vi "Tosca-Test for End of Block.vi"(0 "Result":T1, 1 "SCL in":T2[](array[typedef]), 2 "StimCon Element":T2, 9 "sclIndex":i32, 11 "error in (no error)":errorcluster, 12 "Ncomplete":i32, 13 "Abort":bool) -> (3 "SCL out":T2[](array[typedef]), 4 "Result thru":T1, 6 "End block?":bool, 8 "Abort?":bool, 14 "Ncomplete out":i32, 15 "error out":errorcluster)   [LabVIEW 2020]
uses:
  Typedefs/Tosca-SCL Element.ctl
  Typedefs/Tosca-Schedule Mode.ctl
  Typedefs/Tosca-Event Type.ctl
  Typedefs/Tosca-Trial Result Enum.ctl
  Tosca-Globals.vi
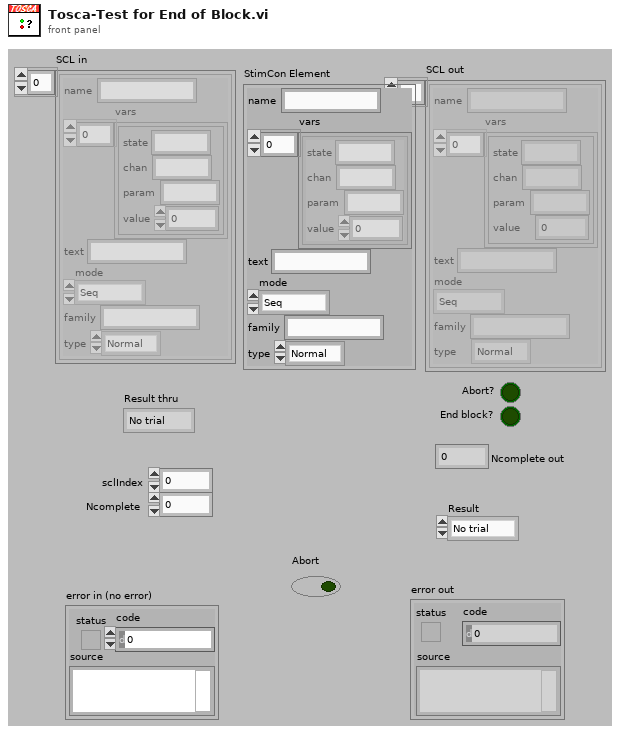
[diagram p1: front panel]
types:
  T1 = typedef "Tosca-Trial Result Enum.ctl" = enum16{"No trial", "Go", "No go", "Error", "Abort"}
  T2 = typedef "Tosca-SCL Element.ctl" = cluster{"name":string, "vars":cluster{"state":string, "chan":string, "param":string, "value":dbl}[], "text":string, "mode":T3, "family":string, "type":T4}
  T3 = typedef "Tosca-Schedule Mode.ctl" = enum16{"Seq", "CS+/CS-", "Adapt"}
  T4 = typedef "Tosca-Event Type.ctl" = enum16{"Normal", "CS+", "CS-"}
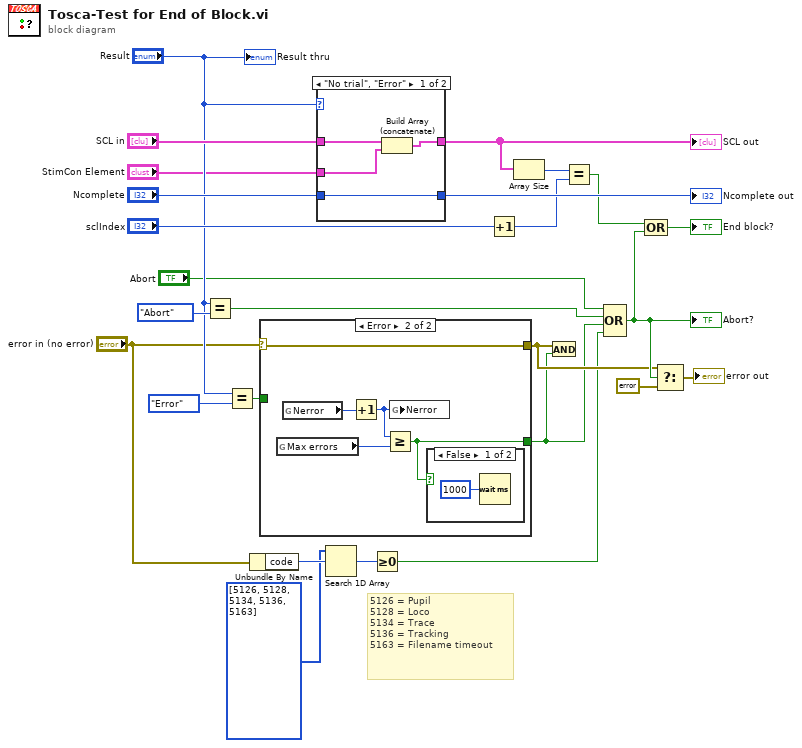
[diagram p0: block diagram]
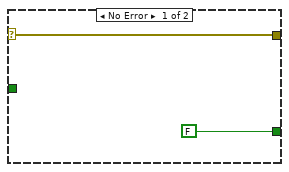
[diagram p2: hidden frame]
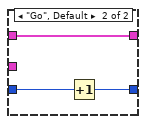
[diagram p4: hidden frame]
diagram:
  # "5126 = Pupil\n5128 = Loco\n5134 = Trace\n5136 = Tracking\n5163 = Filename timeout"
  n1 = Equal?(x="Result", y=Tosca-Trial_Result_Enum."Abort") -> (x = y?=w13:bool)
  n2 = Equal?(x="Result", y=Tosca-Trial_Result_Enum."Error") -> (x = y?=w10:bool)
  n3 = Unbundle By Name("error in (no error)") -> ("code"=w4:i32)
  n4 = case shown="Error" "error in (no error)" {
    selector: "error in (no error)" -> [w27 w29]
    tunnel: [FALSE w30] -> w8
    tunnel: w10 -> [_ _]
    tunnel: [w27 w29] -> w9
    frame No Error {
    }
    frame Error {
      n5 = global read "Tosca-Globals.vi" "Max errors"() -> (w31:i32)
      n6 = global read "Tosca-Globals.vi" "Nerror"() -> (w33:i32)
      n7 = Increment(x=w33) -> (x+1=w32:i32)
      n8 = Greater Or Equal?(x=w32, y=w31) -> (x >= y?=w30:bool)
      n9 = global write "Tosca-Globals.vi" "Nerror"(w32) -> ()
      n10 = case shown="False" w30 {
        frame False {
          n11 = Wait (ms)(milliseconds to wait=u32 1000) -> ()  [unwired: 1 out]
        }
        frame True {
        }
      }
    }
  }
  n12 = case shown="\"No trial\", \"Error\"" "Result" {
    tunnel: "SCL in" -> [w38 w41]
    tunnel: [w36 w41] -> w25
    tunnel: "StimCon Element" -> [w37 _]
    tunnel: "Ncomplete" -> [w35 w40]
    tunnel: [w35 w39] -> w22
    frame "No trial", "Error" {
      n13 = Build Array (concatenate)(w38, w37) -> (w36:T2[])
    }
    frame "Go", Default {
      n14 = Increment(x=w40) -> (x+1=w39:i32)
    }
  }
  "SCL out" <- w25
  "Ncomplete out" <- w22
  n15 = Search 1D Array(1D array=i32[] [5126, 5128, 5134, 5136, 5163], element=w4) -> (index of element=w3:i32)  [unwired: 1 in]
  n16 = Greater Or Equal To 0?(x=w3) -> (x >= 0?=w2:bool)
  n17 = Increment(x="sclIndex") -> (x+1=w18:i32)
  n18 = Array Size(array=w25) -> (size(s)=w20:i32)
  n19 = And(x=w9, y=w8) -> ()  [unwired: 1 out]
  n20 = Equal?(x=w20, y=w18) -> (x = y?=w19:bool)
  n21 = Compound Arithmetic op=OR("Abort", w13, w8, w2) -> (w17:bool)
  "Abort?" <- w17
  n22 = Compound Arithmetic op=OR(w19, w17) -> (→"End block?":bool)
  n23 = Select(t=w9, s=w17, f=errorcluster {"status"=FALSE, "code"=0, "source"=""}) -> (s? t:f=→"error out":errorcluster)
  "Result thru" <- "Result"
